vi "RichToFlatcif_channelcore_ConnectSubscriber.vi"(5 "OutputClusterType":T1, 11 "InputCluster":T2) -> (3 "OutputCluster":T1)   [LabVIEW 2021, in "CIF_Launcher_client.lvlib"]
uses:
  CIF_Launcher_client.lvlib
  cif_channelcore_ConnectSubscriber.ctl
  cif_channelcore_ConnectSubscriber_Flat.ctl
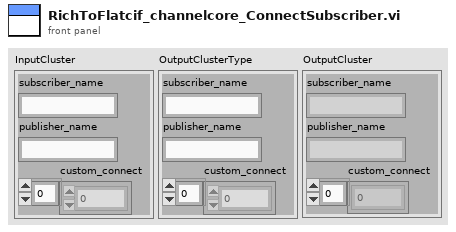
[diagram p1: front panel]
types:
  T1 = typedef "CIF_Launcher_client.lvlib/cif_channelcore_ConnectSubscriber_Flat.ctl" = cluster{"subscriber_name":string, "publisher_name":string, "custom_connect":u8[]}
  T2 = typedef "CIF_Launcher_client.lvlib/cif_channelcore_ConnectSubscriber.ctl" = cluster{"subscriber_name":string, "publisher_name":string, "custom_connect":u8[]}
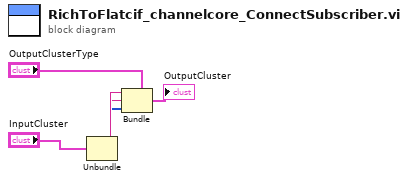
[diagram p0: block diagram]
diagram:
  n1 = Unbundle "Unbundle"("InputCluster") -> ("subscriber_name"=w3:string, "publisher_name"=w2:string, "custom_connect"=w1:u8[])
  n2 = Bundle "Bundle"(cluster="OutputClusterType", "subscriber_name"=w3, "publisher_name"=w2, "custom_connect"=w1) -> (→"OutputCluster":T1)
